vi "NavX Heading.vi"(8 "error in":errorcluster, 11 "Zero Heading?":bool) -> (0 "error out":errorcluster, 2 "Absolute Heading":dbl, 3 "Heading":dbl)   [LabVIEW 2014]
uses:
  Global Objects.vi
  navX Library v2/navX Library v2.lvlib
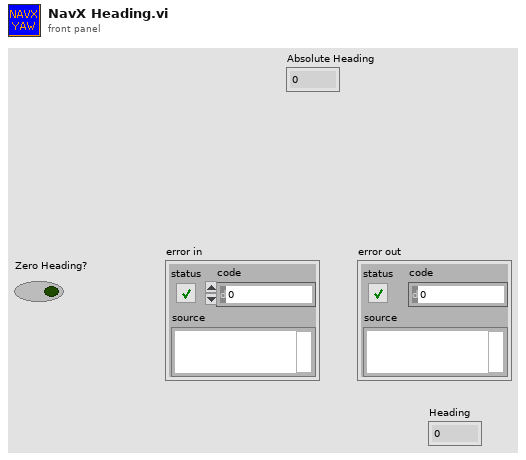
[diagram p1: front panel]
types:
  T1 = typedef "NaxX Info.ctl" = cluster{"navX Device":T2, "Previous Heading":dbl, "Zeroed Heading":dbl}
  T2 = typedef "navX Library v2.lvlib/Z900_navX_DeviceTypeDef.ctl" = cluster{"Interface":cluster{"Protocol":T3, "Update Rate (4Hz-60Hz)":u8, "navX Open TypeDef":variant}, "Notify Packet":refnum<notifier>, "Loop VI Refnum":refnum<vi>, "Ready to Close Occurrence Refnum":refnum<k4>}
  T3 = typedef "navX Library v2.lvlib/Z900_navX_ProtocolTypeDef.ctl" = enum16{"SERIAL", "I2C", "SPI"}
  T4 = cluster{"Yaw":dbl, "Roll":dbl, "Pitch":dbl, "Heading":dbl, "Fused Heading":dbl}
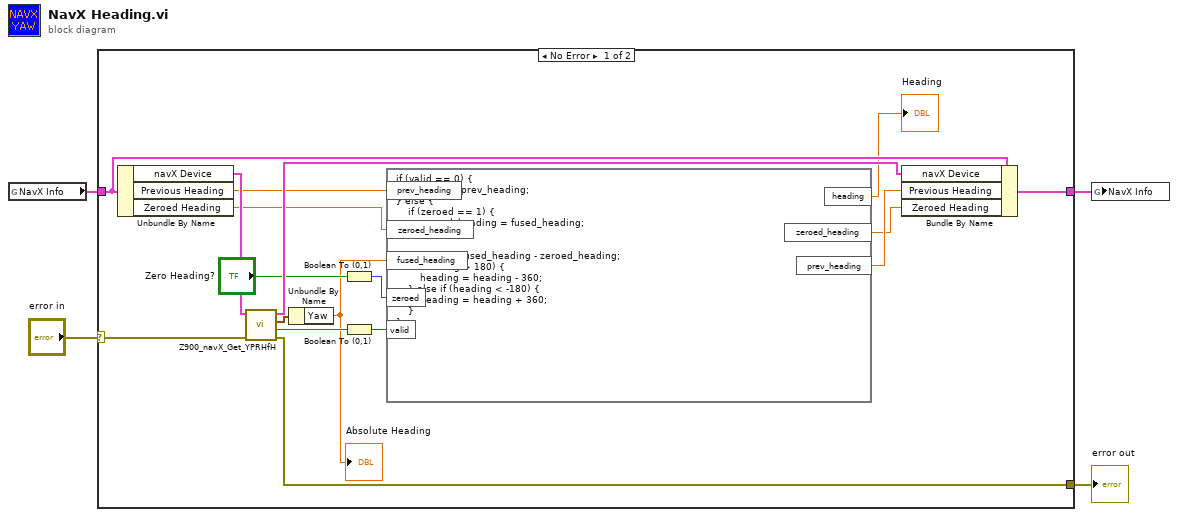
[diagram p0: block diagram]
diagram:
  n1 = global read "Global Objects.vi" "NavX Info"() -> (w2:T1)
  n2 = case shown="No Error" "error in" {
    selector: "error in" -> [w18 w23]
    tunnel: [w17 w23] -> w3
    tunnel: w2 -> [w20 w22]
    tunnel: [w21 w22] -> w1
    frame No Error {
      n3 = Unbundle By Name(w20) -> ("navX Device"=w19:T2, "Previous Heading"=w8:dbl, "Zeroed Heading"=w9:dbl)
      n4 = call "Z900_navX_Get_YPRHfH.vi"("error in (no error)"=w18, "navX Device"=w19) -> ("error out"=w17:errorcluster, "Connected"=w13:bool, "YRPHfH"=w16:T4, "navX Device"=w15:T2)  [unwired: 6 in]
      n5 = Unbundle By Name(w16) -> ("Yaw"=w10:dbl)
      "Absolute Heading" <- w10
      n6 = Boolean To (0,1)(Boolean="Zero Heading?") -> (0, 1=w12:i16)
      n7 = Boolean To (0,1)(Boolean=w13) -> (0, 1=w14:i16)
      n8 = formula code="if (valid == 0) {\n    heading = prev_heading;\n} else {\n    if (zeroed == 1) {\n        zeroed_heading = fused_heading;\n    }\n\n    heading = fused_heading - zeroed_heading;\n    if (heading > 180) {\n        heading = heading - 360;\n    } else if (heading < -180) {\n        heading = heading + 360;\n    }\n}"("prev_heading"=w8, "zeroed_heading"=w9, "fused_heading"=w10, "zeroed"=w12, "valid"=w14) -> ("heading"=→"Heading":dbl, "zeroed_heading"=w6:dbl, "prev_heading"=w7:dbl)
      n9 = Bundle By Name(cluster=w20, "navX Device"=w15, "Previous Heading"=w7, "Zeroed Heading"=w6) -> (w21:T1)
    }
    frame Error {
    }
  }
  "error out" <- w3
  n10 = global write "Global Objects.vi" "NavX Info"(w1) -> ()
